vi "path deletes.vi"(7 "paths in":cluster{cdb, cdb, i32}[](array[cluster]), 11 "new path":bool) -> (8 "path out":cluster{cdb, cdb, i32}[](array[cluster]))   [LabVIEW 2017]
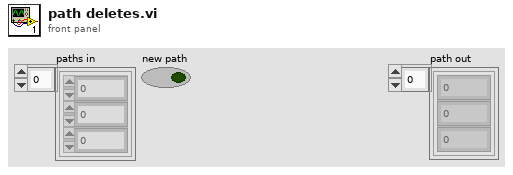
[diagram p1: front panel]
types:
  T1 = cluster{"Numeric":cdb, "Numeric 2":cdb, "Numeric 3":i32}
  T2 = cluster{"Numeric":cdb, "Numeric 2":cdb, "Numeric 3":i32}[]
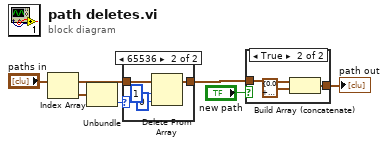
[diagram p0: block diagram]
diagram:
  n1 = Index Array(array="paths in") -> (element=w4:cluster{cdb, cdb, i32})  [unwired: 1 in]
  n2 = Unbundle(w4) -> (w1:i32)  [unwired: 2 out]
  n3 = case shown="65536" w1 {
    tunnel: "paths in" -> [w7 w11]
    tunnel: [w7 w10] -> w2
    frame Default {
    }
    frame 65536 {
      n4 = Delete From Array(array=w11, length=1, index=0) -> (array with subset deleted=w10:cluster{cdb, cdb, i32}[])  [unwired: 1 out]
    }
  }
  n5 = case shown="True" "new path" {
    tunnel: [w12 w14] -> w6
    tunnel: w2 -> [w12 w13]
    frame False {
    }
    frame True {
      n6 = Build Array (concatenate)(w13, T1 {"Numeric"=0.0+0.0i, "Numeric 2"=0.0+0.0i, "Numeric 3"=1} ("Cluster")) -> (w14:T2)
    }
  }
  "path out" <- w6
